vi "Format DataCol.vi"(10 "Data Format":u16(ring) caption="数据格式" items=["十六进制", "十进制", "二进制", "ASCII码"], 11 "Data":T1 {"Direction" items=["Tx", "Rx"]; "CANType" items=["CAN", "CANFD", "CANFD加速"]}) -> (3 "ID str":string)   [LabVIEW 2011, in "CAN FD.lvlib"]
uses:
  CAN FD.lvlib
  Typedef/CAN Data.ctl
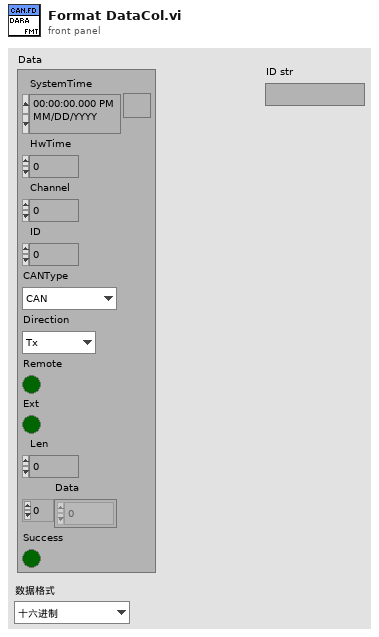
[diagram p1: front panel]
types:
  T1 = typedef "CAN FD.lvlib/CAN Data.ctl" = cluster{"SystemTime":timestamp, "HwTime":dbl, "Channel":u8, "ID":u32, "CANType":i16, "Direction":i16, "Remote":bool, "Ext":bool, "Len":u8, "Data":u8[], "Success":bool}
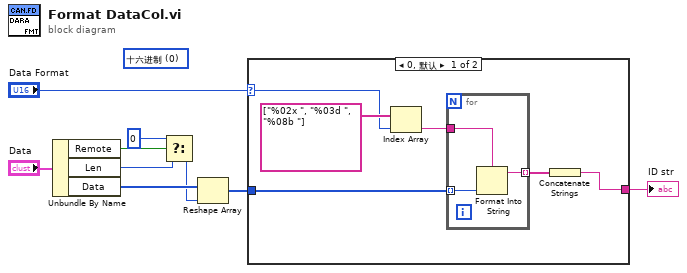
[diagram p0: block diagram]
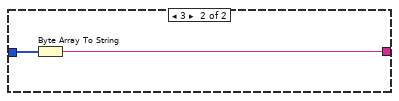
[diagram p2: hidden frame]
diagram:
  (unwired) u16 0 items=["十六进制", "十进制", "二进制", "ASCII码"] ("Data Format")
  n1 = Unbundle By Name("Data") -> ("Remote"=w8:bool, "Len"=w7:u8, "Data"=w6:u8[])
  n2 = Select(t=u8 0, s=w8, f=w7) -> (s? t:f=w5:u8)
  n3 = Reshape Array(w6, w5) -> (w4:u8[])
  n4 = case shown="0, 默认" "Data Format" {
    selector: "Data Format" -> [w14 _]
    tunnel: w4 -> [w13 w20]
    tunnel: [w10 w19] -> w1
    frame 0, Default {
      n5 = Index Array(array=string[] ["%02x ", "%03d ", "%08b "], index=w14) -> (element=w12:string)
      n6 = for {
        tunnel: w13 -> [w18] mode=indexing
        tunnel: w12 -> [w17]
        tunnel: [w16] -> w11 mode=indexing
        n7 = Format Into String(format string=w17, w18) -> (resulting string=w16:string)  [unwired: 2 in, 1 out]
      }
      n8 = Concatenate Strings(w11) -> (w10:string)
    }
    frame 3 {
      n9 = Byte Array To String(unsigned byte array=w20) -> (string=w19:string)
    }
  }
  "ID str" <- w1
